vi "ICNC Set Torch Down Params.vi"(0 "ToolNumber":u32, 1 "ProbingMarginZ":u32, 2 "ProbingSpeedZ":u32, 3 "ProbeInputNumber":u32, 5 "OriginZ":u32, 7 "HeadUpZ":u32, 9 "ProbeTorchOffsetZ":u32, 11 "error in (no error)":errorcluster caption="entrée d'erreur (pas d'erreur)", 12 "FastSpeedDownZ":u32, 13 "FastSpeedUpZ":u32, 14 "ProbeInputState":u32) -> (4 "function return":u32, 15 "error out":errorcluster caption="sortie d'erreur")   [LabVIEW 2012, in "ICNC2.lvlib"]
doc: "DWORD ICNC_SetTorchDownParams(DWORD ToolNumber,\n DWORD OriginZ,\n DWORD HeadUpZ,\n DWORD ProbeTorchOffsetZ,\n DWORD ProbingMarginZ,\n\n DWORD FastSpeedDownZ,\n DWORD ProbingSpeedZ,\n DWORD FastSpeedUpZ,\n DWORD ProbeInputNumber,\n DWORD ProbeInputState);"
uses:
  <userlib>/ICNC/ICNC2.lvlib
  <userlib>/ICNC/ICNC2.dll
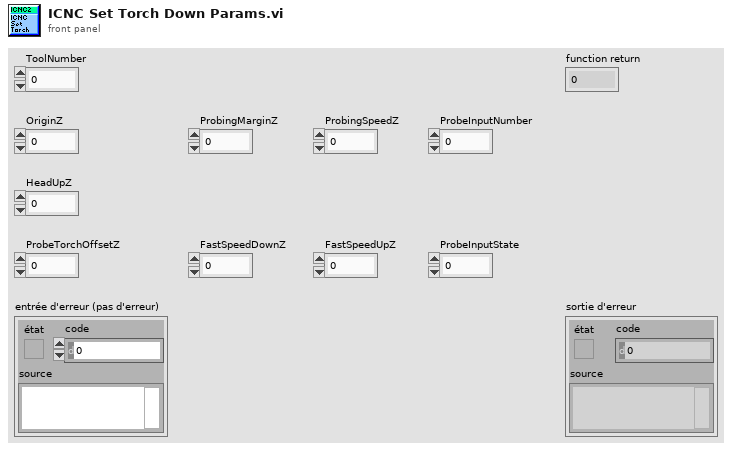
[diagram p1: front panel]
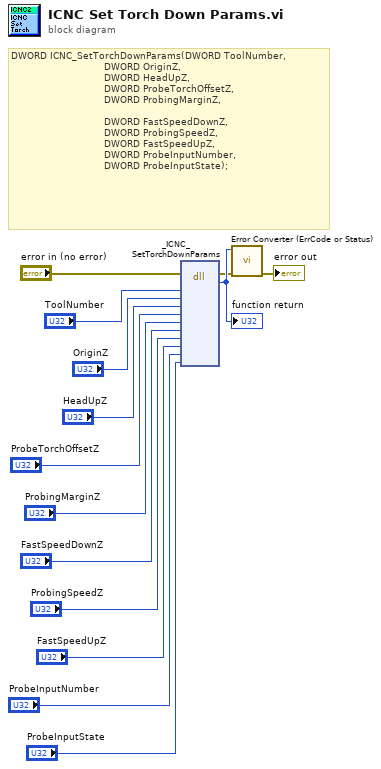
[diagram p0: block diagram]
diagram:
  # "DWORD ICNC_SetTorchDownParams(DWORD ToolNumber,\n                               DWORD OriginZ,\n                               DWORD HeadUpZ,\n                               DWORD ProbeTorchOffsetZ,\n                               DWORD ProbingMarginZ,\n\n                               DWORD FastSpeedDownZ,\n                               DWORD ProbingSpeedZ,\n                               DWORD FastSpeedUpZ,\n                               DWORD ProbeInputNumber,\n                               DWORD ProbeInputState);"
  n1 = dll-call lib="C:/Program Files (x86)/National Instruments/LabVIEW 2012/user.lib/ICNC/ICNC2.*" fn="_ICNC_SetTorchDownParams"(error in="error in (no error)", "ToolNumber"="ToolNumber", "OriginZ"="OriginZ", "HeadUpZ"="HeadUpZ", "ProbeTorchOffsetZ"="ProbeTorchOffsetZ", "ProbingMarginZ"="ProbingMarginZ", "FastSpeedDownZ"="FastSpeedDownZ", "ProbingSpeedZ"="ProbingSpeedZ", "FastSpeedUpZ"="FastSpeedUpZ", "ProbeInputNumber"="ProbeInputNumber", "ProbeInputState"="ProbeInputState") -> (error out=w2:errorcluster, w14:u32)  [unwired: 12 in, 1 out]
  "function return" <- w14
  n2 = call <userlib>:"Error Converter (ErrCode or Status).vi"("error in (no error)"=w2, "error code"=w14) -> ("error out"=→"error out":errorcluster)  [unwired: 9 in]
